vi "Write Multi Binary as Value.vi"(8 "error in (no error)":errorcluster, 9 "Binary":string[](array[string]), 10 "Tag":string[](array[string]), 11 "Var Bus in":refnum<class "Omni_Bus.lvclass">) -> (0 "error out":errorcluster, 3 "Var Bus out":refnum<class "Omni_Bus.lvclass">)   [LabVIEW 2021, in "Omni_Bus.lvclass"]
uses:
  Omni_Bus.lvclass
  Omni_Bus.lvclass/Omni_Bus.ctl
  <vilib>/TSA/Abstract Data Classes/Abs_Types/Value/Abs_Value.lvclass
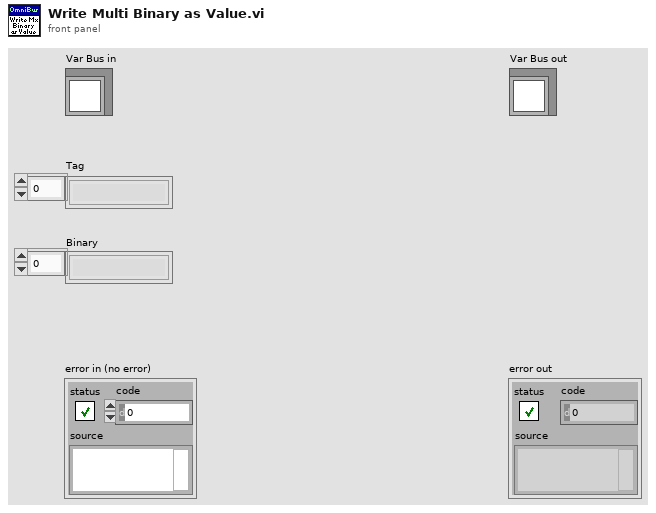
[diagram p1: front panel]
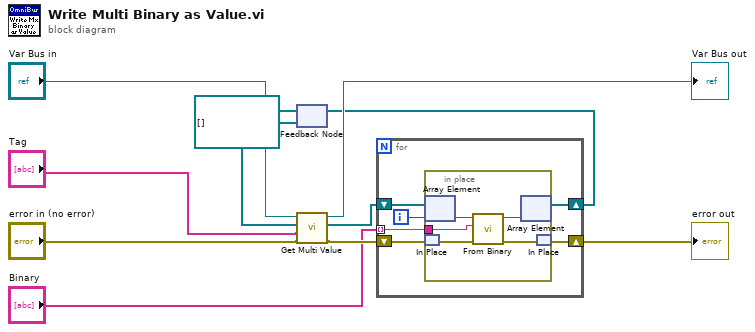
[diagram p0: block diagram]
diagram:
  n1 = feedback #1(refnum<class "Abs_Value.lvclass">[] []) -> (w9:refnum<class "Abs_Value.lvclass">[])
  n2 = call-dynamic "Get Multi Value.vi"("error in (no error)"="error in (no error)", "Tag"="Tag", "Value Type"=w9, "Var Bus in"="Var Bus in") -> ("error out"=w5:errorcluster, "Value Out"=w3:refnum<class "Abs_Value.lvclass">[], "Var Bus out"=→"Var Bus out":refnum<class "Omni_Bus.lvclass">)  [unwired: 5 in]
  n3 = for {
    tunnel: "Binary" -> [w17] mode=indexing
    shift-right: [w12] -> w1
    shift-left: w5 -> [w13]
    shift-right: [w15] -> w2
    shift-left: w3 -> [w16]
    i -> [w14]
    n4 = in-place {
      in-place-border: w17 -> [w18]
      n5 = in-place-array #2(w16, w14) -> (w22:refnum<class "Abs_Value.lvclass">)
      n6 = in-place-match #3(w13) -> (w20:errorcluster)
      n7 = call-dynamic "From Binary.vi"("error in (no error)"=w20, "Binary"=w18, "Type in"=w22) -> ("error out"=w19:errorcluster, "Type out"=w21:refnum<class "Abs_Value.lvclass">)  [unwired: 6 in, 1 out]
      n8 = in-place-array #2(w21) -> (w15:refnum<class "Abs_Value.lvclass">[])  [unwired: 1 out]
      n9 = in-place-match #3(w19) -> (w12:errorcluster)
    }
  }
  "error out" <- w1
  n10 = feedback-in #1(w2) -> ()
